vi "Enable Engine Runno.vi"(6 "error in":errorcluster, 9 "Channel in":u16) -> (0 "error out":errorcluster, 2 "Pass":bool, 3 "Channel out":u16)   [LabVIEW 2023]
uses:
  Communication/PCAN2023/PCAN API.lvlib
panel:
  out "Numeric":i32
  in  "stop 1":bool
  out "MessageBuffer out":T1 {"ID" format="%.0x"; "DATA[0]" format="%.0x"; "DATA[1]" format="%.0x"; "DATA[2]" format="%.0x"; "DATA[3]" format="%.0x"; "DATA[4]" format="%.0x"; "DATA[5]" format="%.0x"; "DATA[6]" format="%.0x"; "DATA[7]" format="%.0x"}
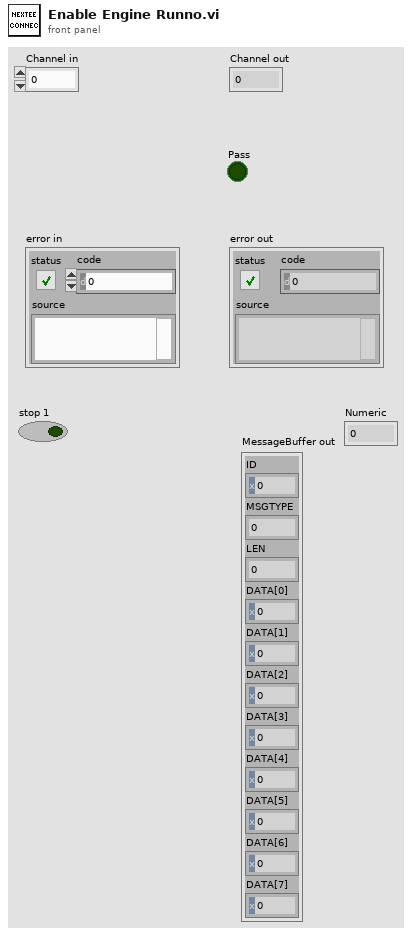
[diagram p1: front panel]
types:
  T1 = cluster{"ID":u32, "MSGTYPE":u8, "LEN":u8, "DATA[0]":u8, "DATA[1]":u8, "DATA[2]":u8, "DATA[3]":u8, "DATA[4]":u8, "DATA[5]":u8, "DATA[6]":u8, "DATA[7]":u8}
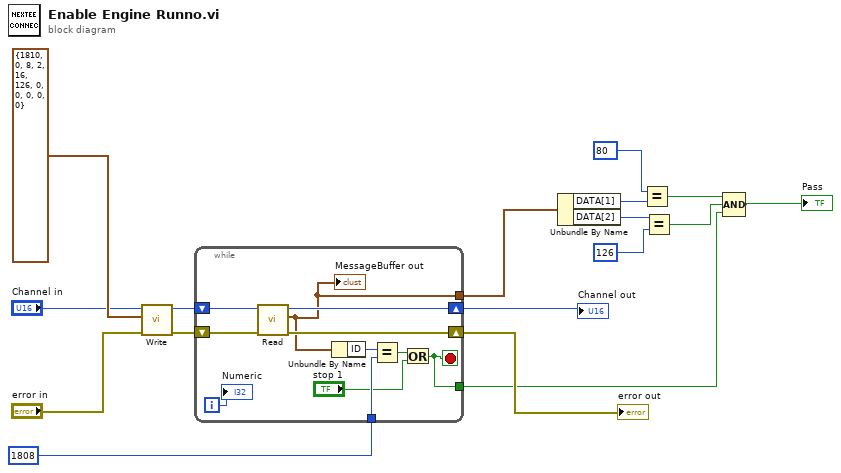
[diagram p0: block diagram]
diagram:
  n1 = call "Write.vi"("error in"="error in", "MessageBuffer"=T1 {"ID"=1810, "MSGTYPE"=0, "LEN"=8, "DATA[0]"=2, "DATA[1]"=16, "DATA[2]"=126, "DATA[3]"=0, "DATA[4]"=0, "DATA[5]"=0, "DATA[6]"=0, "DATA[7]"=0}, "Channel"="Channel in") -> ("error out"=w16:errorcluster, "Channel out"=w15:u16)  [unwired: 5 in, 2 out]
  n2 = while {
    shift-right: [w25] -> w10
    shift-left: w16 -> [w28]
    shift-right: [w26] -> w11
    shift-left: w15 -> [w27]
    tunnel: u32 1808 ("ID") -> [w23]
    tunnel: [w19] -> w9
    tunnel: [w18] -> w4
    i -> [w20]
    stop <- w18 stop-if-true
    n3 = call "Read.vi"("error in"=w28, "Channel"=w27) -> ("error out"=w25:errorcluster, "MessageBuffer out"=w19:T1, "Channel out"=w26:u16)  [unwired: 6 in, 1 out]
    "MessageBuffer out" <- w19
    n4 = Unbundle By Name(w19) -> ("ID"=w24:u32)
    n5 = Equal?(x=w24, y=w23) -> (x = y?=w22:bool)
    n6 = Or(x=w22, y="stop 1") -> (x .or. y?=w18:bool)
    "Numeric" <- w20
  }
  "error out" <- w10
  "Channel out" <- w11
  n7 = Unbundle By Name(w9) -> ("DATA[1]"=w8:u8, "DATA[2]"=w6:u8)
  n8 = Equal?(x=u8 80, y=w8) -> (x = y?=w3:bool)
  n9 = Equal?(x=w6, y=u8 126 ("x")) -> (x = y?=w2:bool)
  n10 = Compound Arithmetic op=AND(w3, w2, w4) -> (→"Pass":bool)
